vi "Demo.vi"() -> ()   [LabVIEW 2020]
uses:
  Simulated Serial/Simulated Serial.lvclass
  C:/git/astemes-lmock/sandbox/Examples/Serial/Serial.lvclass/Serial.lvclass
  String Indicator Logger/String Indicator Logger.lvclass
  C:/git/astemes-lmock/sandbox/Examples/Log/Log.lvclass
  Serial Logging Decorator/Serial Logging Decorator.lvclass
  Driver/Driver.lvclass
panel:
  out "Voltage":dbl
  in  "Measure Voltage":bool
  out "Log":string
  # "This VI Demonstrates how the classes are meant to be composed together when used in an application.\nThe creation and configuration of the classes would be handled by a higher level class, or at the main VI.\nOne important thing to notice, is this allows us to very flexibly declare where the output of log should be directed, or turn off turn off logging, at the highest level - with no changes to the driver."
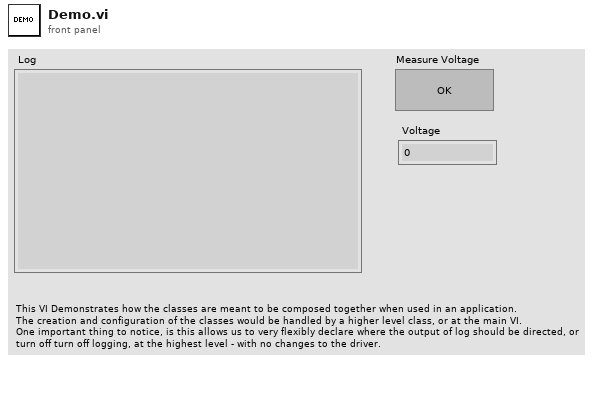
[diagram p1: front panel]
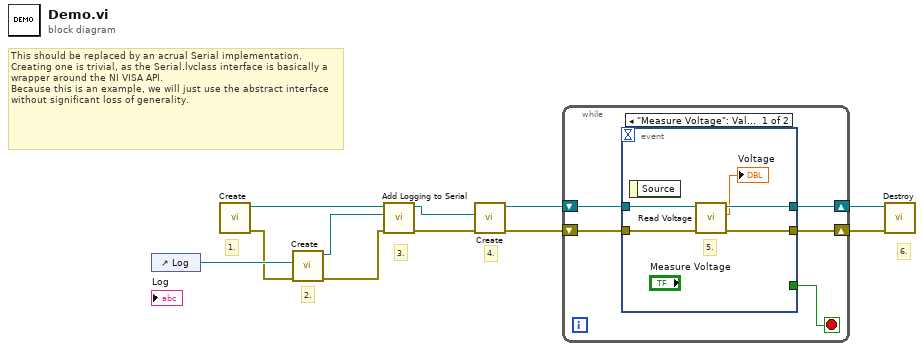
[diagram p0: block diagram]
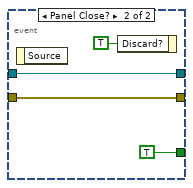
[diagram p2: hidden frame]
diagram:
  # "6."
  # "4."
  # "3."
  # "2."
  # "1."
  # "This should be replaced by an acrual Serial implementation.\nCreating one is trivial, as the Serial.lvclass interface is basically a wrapper around the NI VISA API.\nBecause this is an example, we will just use the abstract interface without significant loss of generality."
  n1 = control-ref of="Log"() -> (w11:refnum<vi>)
  n2 = call "Create.vi"() -> ("error out"=w1:errorcluster, "Simulated Serial"=w2:refnum<class "Simulated Serial.lvclass">)  [unwired: 10 in]
  n3 = call "Create.vi"("error in (no error)"=w1, "Log Reference"=w11) -> ("error out"=w3:errorcluster, "String Indicator Logger"=w10:refnum<class "String Indicator Logger.lvclass">)  [unwired: 8 in]
  n4 = call "Add Logging to Serial.vi"("error in (no error)"=w3, "Log Destination"=w10, "Serial"=w2) -> ("error out"=w8:errorcluster, "Serial with Logging"=w9:refnum<class "Serial.lvclass">)  [unwired: 7 in]
  n5 = call "Create.vi"("error in (no error)"=w8, "Serial"=w9) -> ("error out"=w6:errorcluster, "Driver"=w7:refnum<class "Driver.lvclass">)  [unwired: 8 in]
  n6 = while {
    shift-right: [w14] -> w5
    shift-left: w7 -> [w16]
    shift-right: [w13] -> w4
    shift-left: w6 -> [w15]
    stop <- w12 stop-if-true
    n7 = event shown="[0] \"Measure Voltage\": Value Change" {
      selector: _ -> [_ _]
      dyn-events: _ -> [_ _]
      timeout: _ -> [_ _]
      tunnel: w16 -> [w21 w25]
      tunnel: w15 -> [w20 w24]
      tunnel: [w19 w25] -> w14
      tunnel: [w18 w24] -> w13
      tunnel: [_ TRUE] -> w12
      event "Measure Voltage": Value Change {
        # "5."
        n8 = event-data() -> ()  [unwired: 1 in, 1 out]
        n9 = call "Read Voltage.vi"("error in (no error)"=w20, "Driver In"=w21) -> ("error out"=w18:errorcluster, "Voltage"=→"Voltage":dbl, "Driver Out"=w19:refnum<class "Driver.lvclass">)  [unwired: 7 in]
      }
      event Panel Close? {
        n10 = event-data() -> ()  [unwired: 1 in, 1 out]
        n11 = event-data("Discard?"=TRUE) -> ()  [unwired: 1 in, 1 out]
      }
    }
  }
  n12 = call "Destroy.vi"("error in (no error)"=w4, "Driver"=w5) -> ()  [unwired: 9 in, 1 out]
